vi "CutTest.vi"() -> ()   [LabVIEW 2014]
uses:
  TypeDefs/Point3D.ctl
  <vilib>/picture/3D Picture Control/Object/Create Object (name).vi
  <vilib>/picture/3D Picture Control/NI_3D Picture Control.lvlib
panel:
  out "XY Graph":T1(graph)
  out "error out":errorcluster
  out "NumTriIntersected":i32
  out "3D Picture":refnum<vi>(3d-picture)
  in  "CuttingZ":sgl
  out "Center 2":T2
  out "MaxDims 2":T2
  out "MinDims 2":T2
  in  "STL Path":path
  out "Center":T2
  out "MaxDims":T2
  out "MinDims":T2
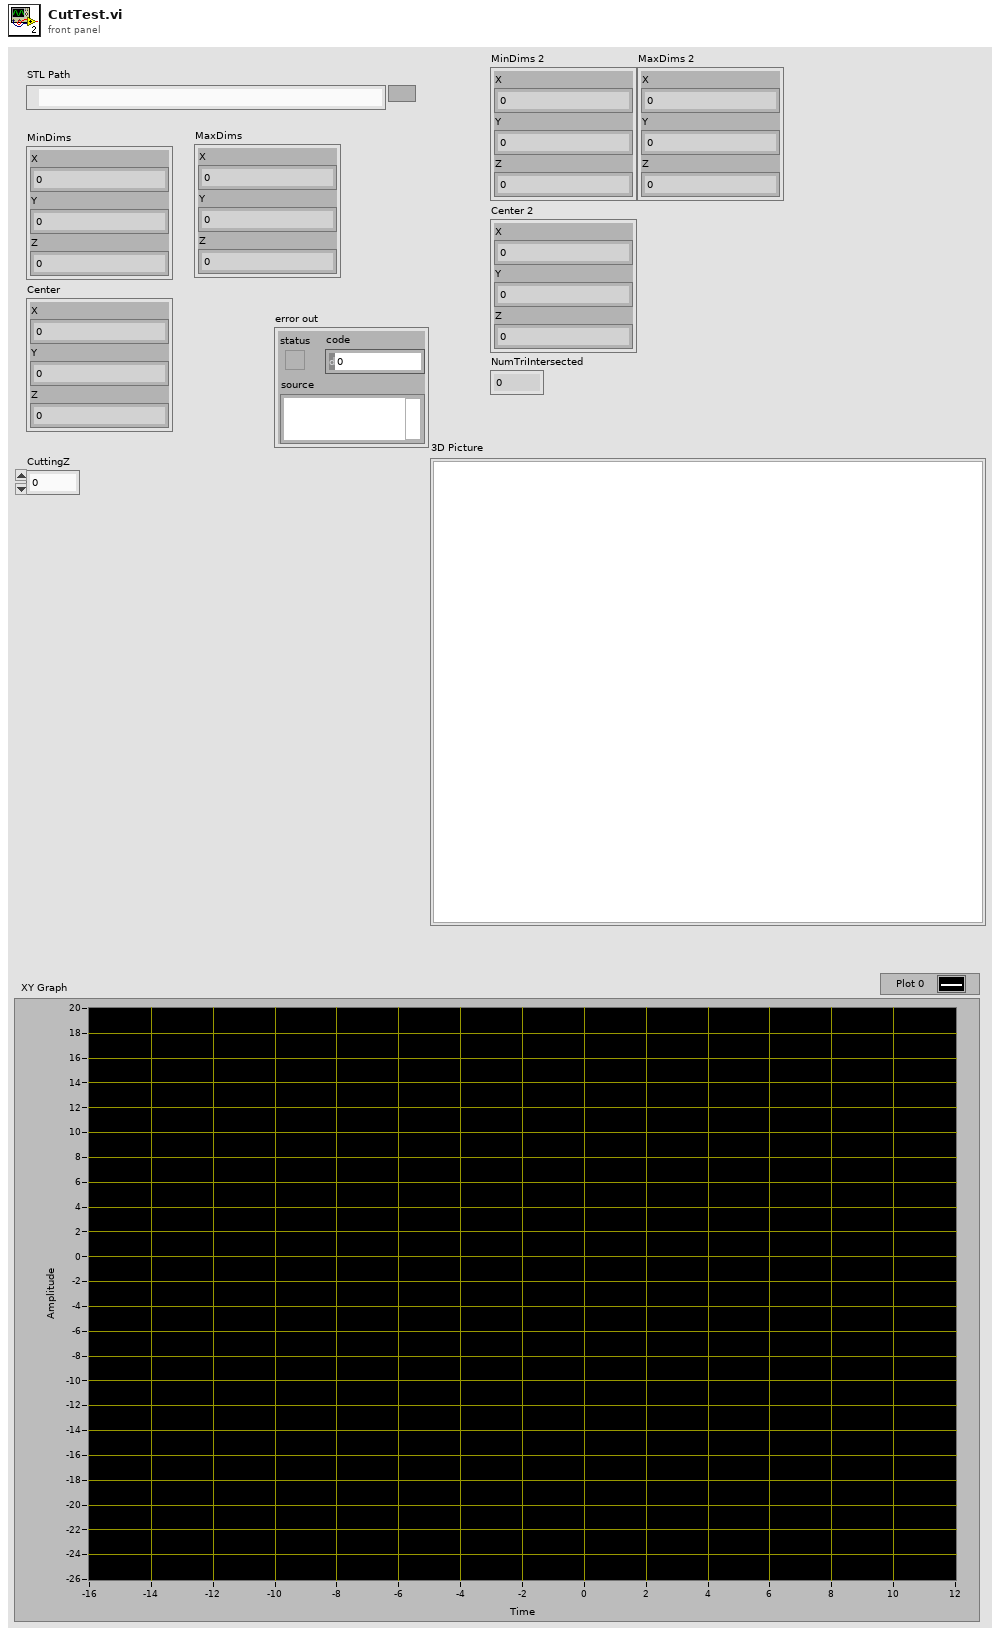
[diagram p1: front panel]
types:
  T1 = cluster{"VertexArray":cluster{"X":sgl, "Y":sgl}[]}[]
  T2 = typedef "Point3D.ctl" = cluster{"X":sgl, "Y":sgl, "Z":sgl}
  T3 = typedef "TriangleFace.ctl" = cluster{"Normal":T2, "Vertex1":T2, "Vertex2":T2, "Vertex3":T2}
  T4 = enum16{"Overall", "Per Primitive", "Per Vertex", "Binding Off"}
  T5 = cluster{"Red":sgl, "Green":sgl, "Blue":sgl, "Alpha":sgl}[]
  T6 = enum16{"Points", "Lines", "Line Strip", "Line Loop", "Triangles", "Triangle Strip", "Triangle Fan", "Quads", "Quad Strip", "Polygon"}
  T7 = typedef "Line2D.ctl" = cluster{"Vertex1":T8, "Vertex2":T8}
  T8 = typedef "Point2D.ctl" = cluster{"X":sgl, "Y":sgl}
  T9 = typedef "Poly2D.ctl" = cluster{"VertexArray":T8[]}
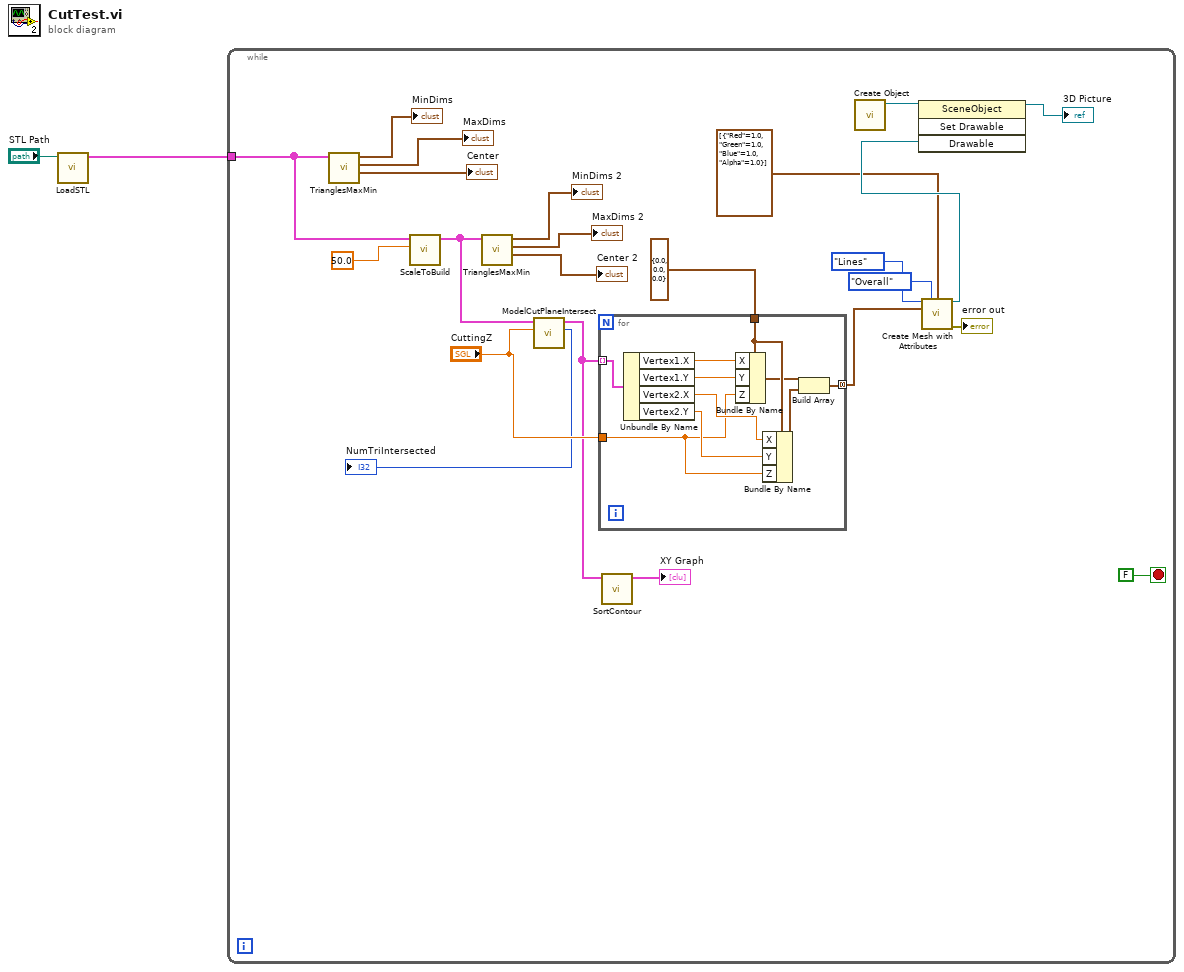
[diagram p0: block diagram]
diagram:
  n1 = call "LoadSTL.vi"("STL Path"="STL Path") -> ("Triangles"=w1:T3[])  [unwired: 8 in, 2 out]
  n2 = while {
    tunnel: w1 -> [w22]
    stop <- FALSE stop-if-true
    n3 = call "TrianglesMaxMin.vi"("Triangles"=w22) -> ("Center"=→"Center":T2, "MaxDims"=→"MaxDims":T2, "MinDims"=→"MinDims":T2)  [unwired: 8 in]
    n4 = call "ScaleToBuild.vi"("BuildSize"=50.0, "Triangles"=w22) -> ("TrianglesOut"=w17:T3[])  [unwired: 9 in]
    n5 = call "TrianglesMaxMin.vi"("Triangles"=w17) -> ("Center"=→"Center 2":T2, "MaxDims"=→"MaxDims 2":T2, "MinDims"=→"MinDims 2":T2)  [unwired: 8 in]
    n6 = call "ModelCutPlaneIntersect.vi"("CuttingZ"="CuttingZ", "Triangles"=w17) -> ("NumTriIntersected"=→"NumTriIntersected":i32, "LineArray"=w4:T7[])  [unwired: 8 in]
    n7 = for {
      tunnel: w4 -> [w35] mode=indexing
      tunnel: cluster{"X":sgl, "Y":sgl, "Z":sgl} {"X"=0.0, "Y"=0.0, "Z"=0.0} ("3D Point") -> [w32]
      tunnel: "CuttingZ" -> [w29]
      tunnel: [w26] -> w5 mode=concatenating
      n8 = Unbundle By Name(w35) -> ("Vertex1.X"=w34:sgl, "Vertex1.Y"=w33:sgl, "Vertex2.X"=w31:sgl, "Vertex2.Y"=w30:sgl)
      n9 = Bundle By Name(cluster=w32, "X"=w34, "Y"=w33, "Z"=w29) -> (w28:cluster{"X":sgl, "Y":sgl, "Z":sgl})
      n10 = Bundle By Name(cluster=w32, "X"=w31, "Y"=w30, "Z"=w29) -> (w27:cluster{"X":sgl, "Y":sgl, "Z":sgl})
      n11 = Build Array(w28, w27) -> (w26:cluster{"X":sgl, "Y":sgl, "Z":sgl}[])
    }
    n12 = call "SortContour.vi"("LineArray"=w4) -> ("Polys"=→"XY Graph":T9[])  [unwired: 10 in]
    n13 = call-poly <vilib>:"Create Object.vi"() -> ("Scene:New Object"=w16:refnum<vi>)  [unwired: 10 in, 1 out]
    n14 = call <vilib>:"Create Mesh with Attributes.vi"("Draw Mode"=T6."Lines", "Color Binding Mode"=T4."Overall", "Color Array"=T5 [{"Red"=1.0, "Green"=1.0, "Blue"=1.0, "Alpha"=1.0}], "Vertex Array"=w5) -> ("New Mesh Refnum"=w12:refnum<vi>, "error out"=→"error out":errorcluster)  [unwired: 10 in]
    n15 = invoke class="SceneObject" method="Set Drawable"(reference=w16, "Drawable"=w12) -> (reference out=→"3D Picture":refnum<vi>)  [unwired: 2 in, 3 out]
  }
